vi "Launch Helper Main.vi"(8 "error in":errorcluster) -> (0 "error out":errorcluster, 2 "Events":T1, 3 "Controls":T2(array[cluster]))   [LabVIEW 2020, in "Test.Maui 2.0.Panels.lvclass"]
uses:
  Test.Maui 2.0.Panels/Test.Maui 2.0.Panels.lvclass
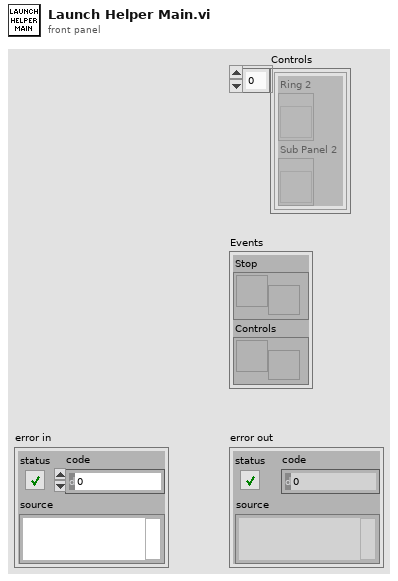
[diagram p1: front panel]
types:
  T1 = cluster{"Stop":refnum<user-event>, "Controls":refnum<user-event>}
  T2 = cluster{"Ring 2":refnum<vi>, "Sub Panel 2":refnum<vi>}[]
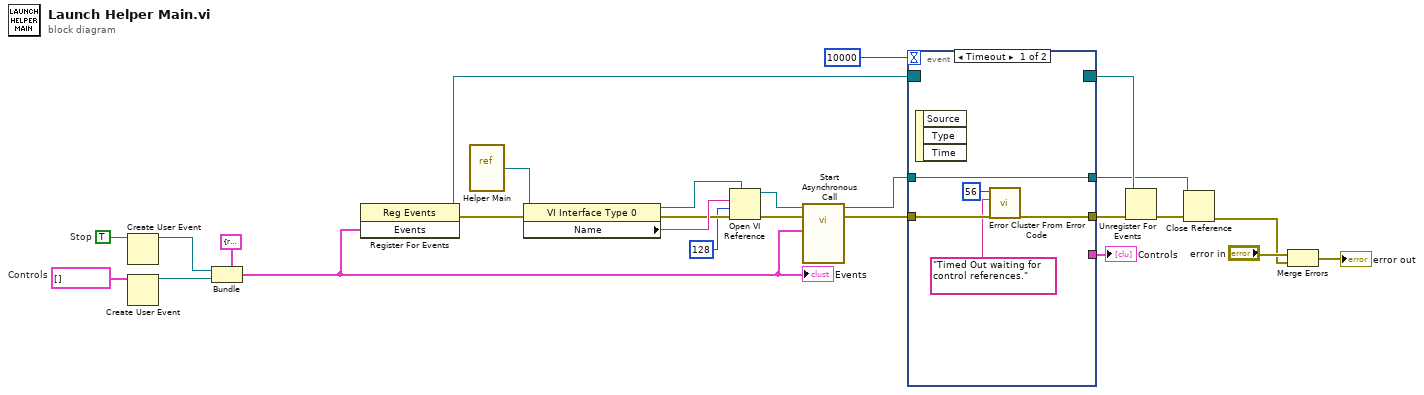
[diagram p0: block diagram]
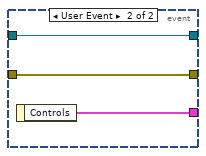
[diagram p2: hidden frame]
diagram:
  w23 = TRUE  # Stop
  w26 = T2 []  # Controls
  n1 = Create User Event(user event datatype=w23) -> (user event=w24:refnum<user-event>)  [unwired: 1 in, 1 out]
  n2 = Create User Event(user event datatype=w26) -> (user event=w25:refnum<user-event>)  [unwired: 1 in, 1 out]
  n3 = Bundle(cluster=T1 {"Stop"=refnum, "Controls"=refnum} ("Events"), "Stop"=w24, "Controls"=w25) -> (w4:T1)
  "Events" <- w4
  n4 = register-events(w4) -> (reference out=w17:refnum<event-registration>, error out=w21:errorcluster)  [unwired: 2 in]
  n5 = vi-ref "Helper Main.vi"() -> (w3:refnum<vi>)
  n6 = property class="VI Interface Type 0"(reference=w3, error in=w21) -> (reference out=w1:refnum<vi>, error out=w20:errorcluster, "Name"=w22:string)
  n7 = Open VI Reference(type specifier VI Refnum (for type only)=w1, vi path=w22, options=128, error in (no error)=w20) -> (vi reference=w18:refnum<vi>, error out=w19:errorcluster)  [unwired: 2 in]
  n8 = call-by-ref "Start Asynchronous Call"(reference=w18, error in=w19, "Events"=w4) -> (reference out=w15:refnum<vi>, error out=w16:errorcluster)  [unwired: 11 in]
  n9 = event shown="[0] Timeout" {
    selector: w17 -> [_ _]
    dyn-events: [_ _] -> w14
    timeout: 10000 -> [_ _]
    tunnel: w16 -> [w29 w34]
    tunnel: w15 -> [w31 w33]
    tunnel: [w30 w34] -> w13
    tunnel: [w31 w33] -> w11
    tunnel: [_ w32] -> w8
    event Timeout {
      n10 = event-data() -> ()  [unwired: 1 in, 3 out]
      n11 = call <vilib>:"Error Cluster From Error Code.vi"("error in (no error)"=w29, "error message (\"\")"="Timed Out waiting for control references." ("error message (\"\")"), "error code (0)"=56) -> ("error out"=w30:errorcluster)  [unwired: 6 in]
    }
    event User Event {
      n12 = event-data() -> ("Controls"=w32:T2)  [unwired: 1 in]
    }
  }
  "Controls" <- w8
  n13 = Unregister For Events(event registration refnum=w14, error in=w13) -> (error out=w12:errorcluster)
  n14 = Close Reference(reference=w11, error in (no error)=w12) -> (error out=w6:errorcluster)
  n15 = Merge Errors("error in", w6) -> (→"error out":errorcluster)
